vi "Write Robodolf Controller State.vi"(8 "error in (no error)":errorcluster, 10 "Controller State":T1, 11 "RDS State in":refnum<class "RDS State.lvclass">) -> (0 "error out":errorcluster, 3 "RDS State out":refnum<class "RDS State.lvclass">)   [LabVIEW 2015, in "RDS Child Messages.lvlib" / "RDS State.lvclass"]
uses:
  RDS State.lvclass
  Actors/RDS Controller Actor/RDS Controller Actor/Controller.ctl
  RDS State.lvclass/RDS State.ctl
  Actors/RDS Controller Actor/RDS Controller Actor/RDS Controller Actor.lvlib
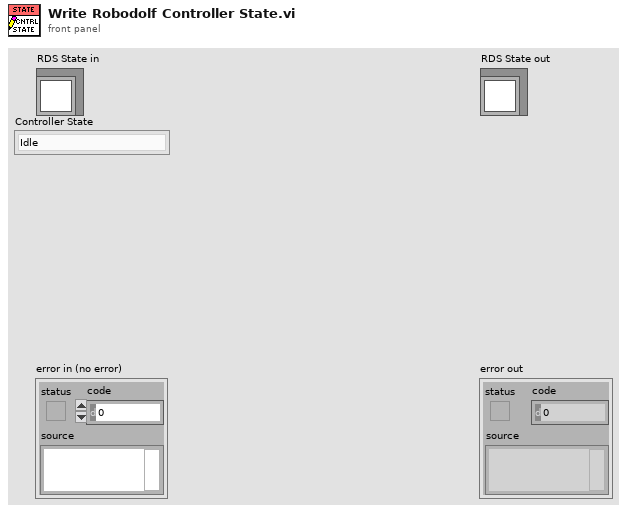
[diagram p1: front panel]
types:
  T1 = typedef "RDS Controller Actor.lvlib/Controller.ctl" = enum16{"Idle", "Local Remote Control", "Shore Remote Control", "Mission Control"}
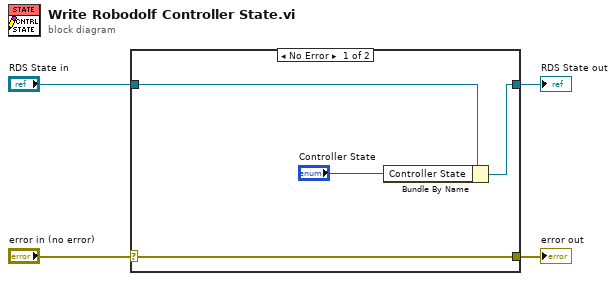
[diagram p0: block diagram]
diagram:
  n1 = case shown="No Error" "error in (no error)" {
    selector: "error in (no error)" -> [w8 w9]
    tunnel: [w8 w9] -> w3
    tunnel: [w6 w10] -> w1
    tunnel: "RDS State in" -> [w7 w10]
    frame No Error {
      n2 = Bundle By Name(cluster=w7, "Controller State"="Controller State") -> (w6:refnum<class "RDS State.lvclass">)
    }
    frame Error {
    }
  }
  "error out" <- w3
  "RDS State out" <- w1
